vi "Py.vi"() -> ()   [LabVIEW 2024]
panel:
  out "return value":dbl
  in  "Array":dbl[](array[numeric])
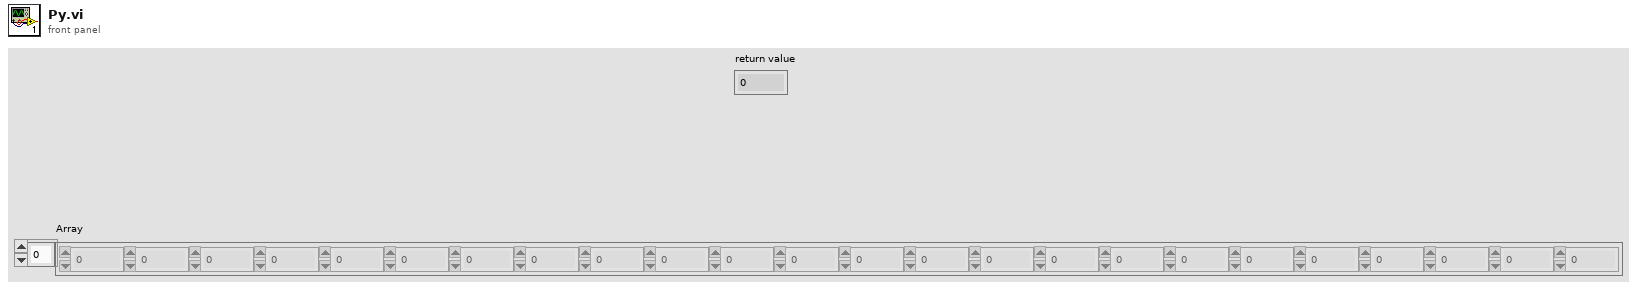
[diagram p1: front panel]
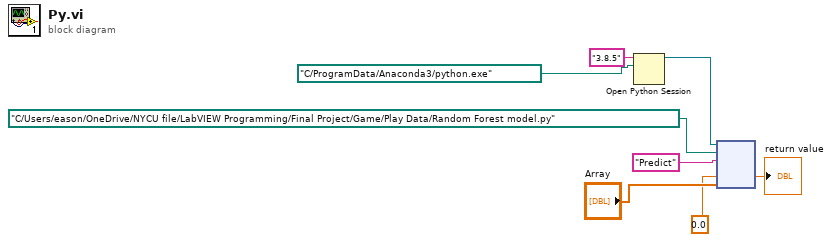
[diagram p0: block diagram]
diagram:
  n1 = Open Python Session(python version="3.8.5" ("Python version"), python path=path "C:/ProgramData/Anaconda3/python.exe" ("Python path")) -> (session out=w5:refnum<k35>)  [unwired: 1 in, 1 out]
  n2 = node(w5, path "C:/Users/eason/OneDrive/NYCU file/LabVIEW Programming/Final Project/Game/Play Data/Random Forest model.py" ("module path"), "Predict" ("function name"), 0.0, "Array") -> (→"return value":dbl)  [unwired: 2 in, 4 out]
